vi "Write Configuration Data.vi"(0 "Lock-In Variable Channels in":refnum<class "Lock-In Variable Channels_2.lvclass">, 1 "AO Configuration Control":T3(array[cluster]), 3 "AI Configuration Control":T4(array[cluster])=[{"AI.Coupling"=10050, "AI.Max"=10.0, "AI.Min"=-10.0, "Input physical channels"="PXI1Slot2/ai0:1"}, {"AI.Coupling"=10050, "AI.Max"=10.0, "AI.Min"=-10.0, "Input physical channels"="PXI1Slot3/ai0:1"}, {"AI.Coupling"=10050, "AI.Max"=10.0, "AI.Min"=-10.0, "Input physical channels"="PXI1Slot6/ai0:1"}] {"AI.Coupling" items=["AC"=10045, "DC"=10050, "GND"=10066]}, 4 "AI Block Size Control":i32, 5 "AI Buffer Size (s) Control":i32, 7 "error in (no error)":errorcluster, 8 "Max AI Rate Control":i32, 9 "Auto Control Max AI Rate/AI Block Size Control":bool, 10 "Phase&Tc Control":T1(array[cluster]), 11 "Input Signals Control":i16, 12 "OSC Configuration Control":T2(array[cluster])) -> (20 "Lock-In Variable Channels out":refnum<class "Lock-In Variable Channels_2.lvclass">, 27 "error out":errorcluster)   [LabVIEW 2011, in "Lock-In Variable Channels_2.lvclass"]
uses:
  Lock-In Variable Channels_2.lvclass
  Lock-In Variable Channels_2.lvclass/Lock-In Variable Channels_2.ctl
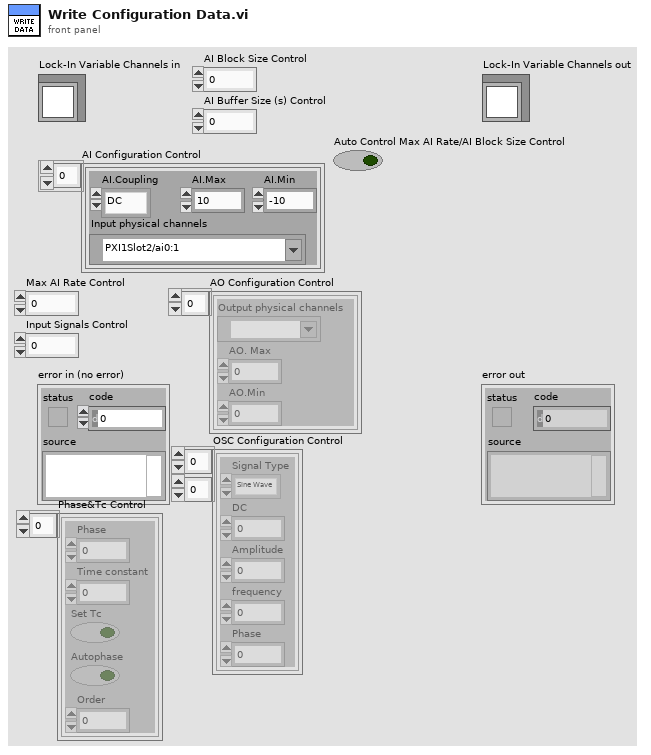
[diagram p1: front panel]
types:
  T1 = cluster{"Phase":dbl, "Time constant":dbl, "Set Tc":bool, "Autophase":bool, "Order":dbl}[]
  T2 = cluster{"Signal Type":enum16{"Sine Wave", "Triangle Wave", "Square Wave", "Sawtooth Wave"}, "DC":dbl, "Amplitude":dbl, "frequency":dbl, "Phase":dbl}[][]
  T3 = cluster{"Output physical channels":tag, "AO. Max":dbl, "AO.Min":dbl}[]
  T4 = cluster{"AI.Coupling":i32, "AI.Max":dbl, "AI.Min":dbl, "Input physical channels":tag}[]
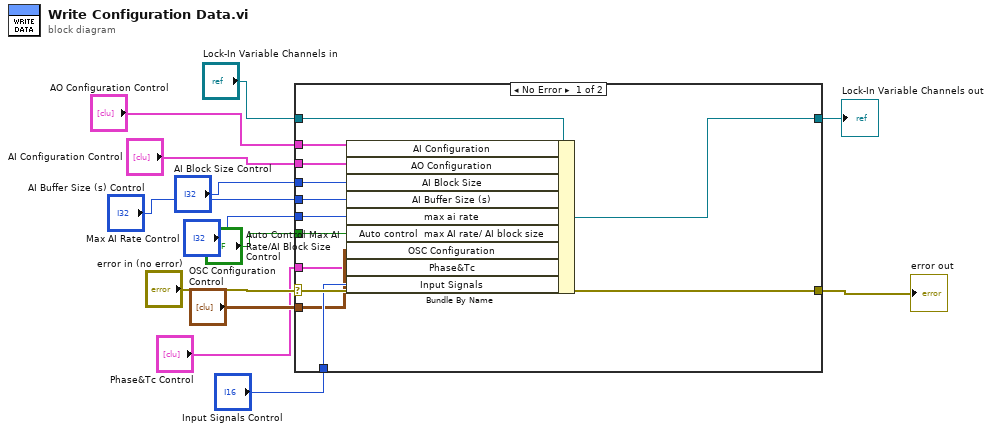
[diagram p0: block diagram]
diagram:
  n1 = case shown="No Error" "error in (no error)" {
    selector: "error in (no error)" -> [w25 w26]
    tunnel: [w25 w26] -> w12
    tunnel: [w23 w27] -> w10
    tunnel: "Lock-In Variable Channels in" -> [w24 w27]
    tunnel: "AI Configuration Control" -> [w22 _]
    tunnel: "AO Configuration Control" -> [w21 _]
    tunnel: "AI Block Size Control" -> [w20 _]
    tunnel: "AI Buffer Size (s) Control" -> [w19 _]
    tunnel: "Max AI Rate Control" -> [w18 _]
    tunnel: "Auto Control Max AI Rate/AI Block Size Control" -> [w17 _]
    tunnel: "Input Signals Control" -> [w16 _]
    tunnel: "OSC Configuration Control" -> [w15 _]
    tunnel: "Phase&Tc Control" -> [w14 _]
    frame No Error {
      n2 = Bundle By Name(cluster=w24, "AI Configuration"=w22, "AO Configuration"=w21, "AI Block Size"=w20, "AI Buffer Size (s)"=w19, "max ai rate"=w18, "Auto control  max AI rate/ AI block size"=w17, "OSC Configuration"=w15, "Phase&Tc"=w14, "Input Signals"=w16) -> (w23:refnum<class "Lock-In Variable Channels_2.lvclass">)
    }
    frame Error {
    }
  }
  "error out" <- w12
  "Lock-In Variable Channels out" <- w10
